vi "电子学自测试.vi"() -> ()   [LabVIEW 2017]
panel:
  in  "data  path":path=path "G:/rpc测试"
  out "appended path":path=path "D:/rpc测试/test_20260314_040925.txt"
  in  "filename":string="test"
  out "异常板卡":cluster{i32, i32}[](array[cluster])
  out "数字":i32=500
  out "当前累计":bool[][](array[boolean])
  out "当前Middle":bool[][](array[boolean])
  in  "停止":bool
  out "当前TDC":bool[](array[boolean])
  out "最终结果":bool[][][](array[boolean])
  out "trigger_rate":dbl[](array[numeric])=[-1.0, -1.0, -1.0, -1.0, -1.0, -1.0, -1.0, -1.0, -1.0, -1.0]
  out "error out":errorcluster
  out "TDC_ID":u64=2
  out "Middle ID":u64=1
  in  "TriggerRate":u8(ring)=2 items=["125Hz", "250Hz", "500Hz", "1000Hz", "2000Hz", "4000Hz", "5000Hz", "10000Hz", "20000Hz", "50000Hz"]
  in  "SoftTrigger":bool=TRUE
  in  "error in (no error)":errorcluster
  in  "address":string="10.3.173.20"
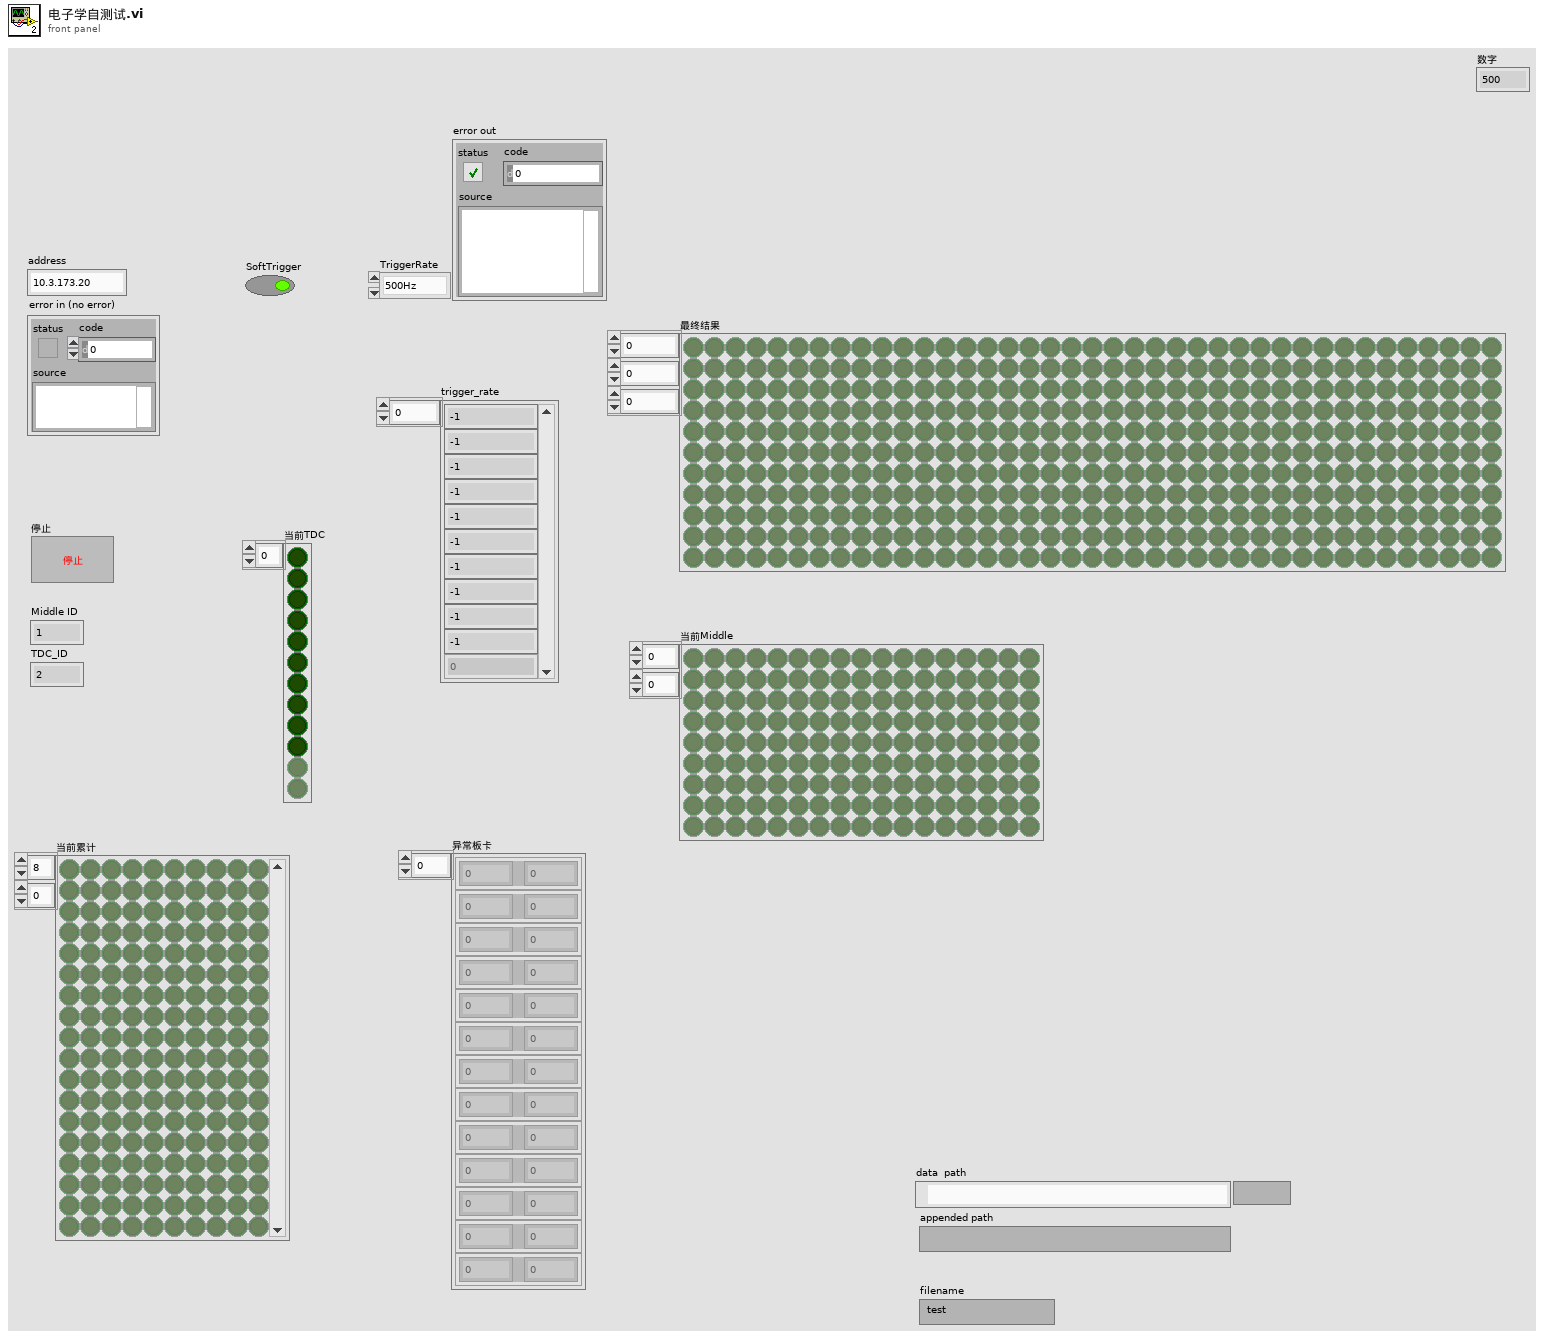
[diagram p1: front panel]
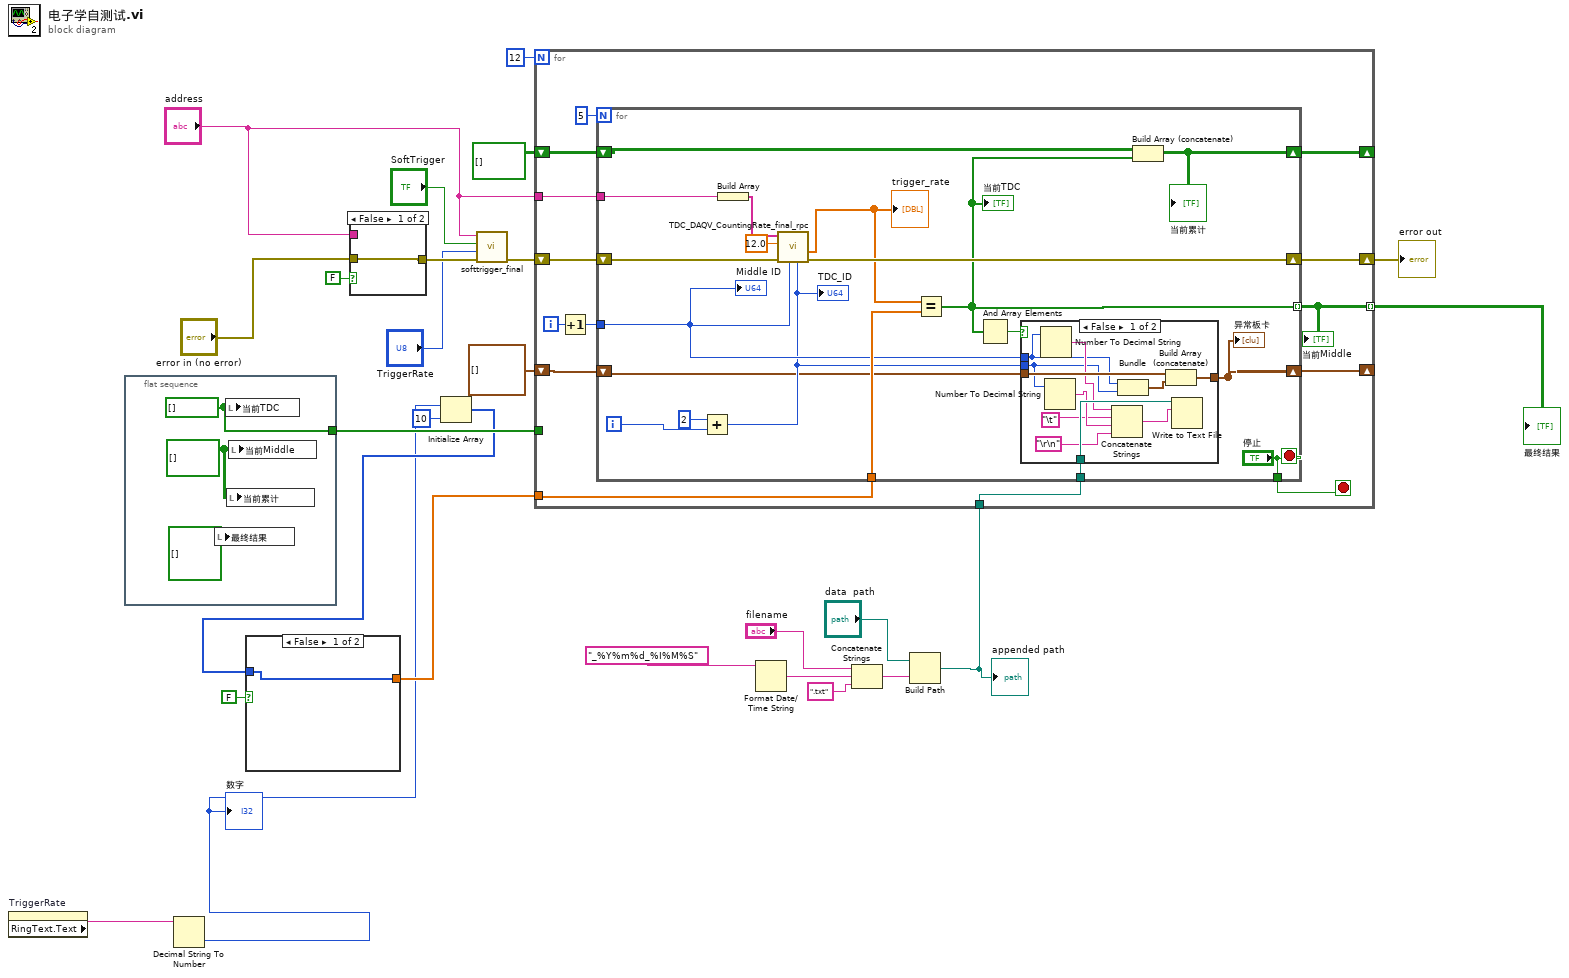
[diagram p0: block diagram]
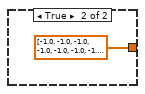
[diagram p2: hidden frame]
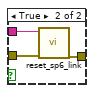
[diagram p4: hidden frame]
diagram:
  n1 = property on="TriggerRate" class="Ring (strict)"() -> ("RingText.Text"=w11:string)  [unwired: 2 in, 2 out]
  n2 = flat-sequence {
    tunnel: [w27] -> w14
    frame #0 {
      w29 = bool[][] [] ("当前Middle")
      w27 = bool[] [] ("当前TDC")
      n3 = local write "最终结果"(bool[][][] [] ("数组")) -> ()
      n4 = local write "当前TDC"(w27) -> ()
      n5 = local write "当前累计"(w29) -> ()
      n6 = local write "当前Middle"(w29) -> ()
    }
  }
  n7 = Decimal String To Number(string=w11) -> (number=w9:i32)  [unwired: 2 in, 1 out]
  "数字" <- w9
  n8 = case shown="False" FALSE {
    tunnel: "error in (no error)" -> [w30 w33]
    tunnel: [w30 w32] -> w25
    tunnel: "address" -> [_ w31]
    frame False {
    }
    frame True {
      n9 = call "reset_sp6_link.vi"("error in (no error)"=w33, "address"=w31) -> ("error out"=w32:errorcluster)  [unwired: 9 in]
    }
  }
  n10 = Initialize Array(w9, 10 ("维数大小")) -> (w12:i32[])
  n11 = case shown="False" FALSE {
    tunnel: [w34 dbl[] [-1.0, -1.0, -1.0, -1.0, -1.0, -1.0, -1.0, -1.0, -1.0, -1.0] ("rate_array")] -> w16
    tunnel: w12 -> [w34 _]
    frame False {
    }
    frame True {
    }
  }
  n12 = call "softtrigger_final.vi"("error in (no error)"=w25, "TriggerRate"="TriggerRate", "SoftTrigger"="SoftTrigger", "address"="address") -> ("error out"=w22:errorcluster)  [unwired: 7 in]
  n13 = Format Date/Time String(time format string (%c)="_%Y%m%d_%I%M%S") -> (date/time string=w6:string)  [unwired: 2 in]
  n14 = Concatenate Strings("filename", w6, ".txt") -> (w8:string)
  n15 = Build Path(base path="data  path", name or relative path=w8) -> (appended path=w3:path)
  "appended path" <- w3
  n16 = for {
    N: 12 -> [_]
    tunnel: "address" -> [w49]
    shift-right: [w47] -> w21
    shift-left: w22 -> [w48]
    tunnel: w16 -> [w45]
    tunnel: [w44] -> w18 mode=indexing
    shift-right: [w40] -> _
    shift-left: bool[][] [] -> [w39]
    tunnel: w14 -> [_]
    shift-right: [w38] -> _
    shift-left: cluster{i32, i32}[] [] -> [w37]
    tunnel: w3 -> [w36]
    i -> [w46]
    stop <- w41 stop-if-true
    n17 = Increment(x=w46) -> (x+1=w42:i32)
    n18 = for {
      N: 5 -> [_]
      tunnel: w49 -> [w68]
      shift-right: [w65] -> w47
      shift-left: w48 -> [w66]
      tunnel: w42 -> [w54]
      tunnel: w45 -> [w62]
      tunnel: [w56] -> w44 mode=indexing
      tunnel: ["停止"] -> w41
      shift-right: [w59] -> w40
      shift-left: w39 -> [w58]
      shift-right: [w50] -> w38
      shift-left: w37 -> [w52]
      tunnel: w36 -> [w51]
      i -> [w64]
      stop <- "停止" stop-if-true
      n19 = Add(x=2, y=w64) -> (x+y=w53:i32)
      "TDC_ID" <- w53
      n20 = Build Array(w68) -> (w67:string[])
      n21 = call "TDC_DAQV_CountingRate_final_rpc.vi"("TDC_ID"=w53, "Middle ID"=w54, "error in (no error)"=w66, "timeout"=12.0, "Array"=w67) -> ("error out"=w65:errorcluster, "trigger_rate"=w63:dbl[])  [unwired: 4 in, 1 out]
      "trigger_rate" <- w63
      n22 = Equal?(x=w63, y=w62) -> (x = y?=w56:bool[])
      "当前TDC" <- w56
      n23 = And Array Elements(Boolean array=w56) -> (logical AND=w55:bool)
      n24 = case shown="False" w55 {
        tunnel: w54 -> [w70 _]
        tunnel: w53 -> [w69 _]
        tunnel: w52 -> [w79 w80]
        tunnel: [w78 w80] -> w50
        tunnel: w51 -> [w76 _]
        frame False {
          n25 = Number To Decimal String(number=w70) -> (decimal integer string=w74:string)  [unwired: 1 in]
          n26 = Number To Decimal String(number=w69) -> (decimal integer string=w73:string)  [unwired: 1 in]
          n27 = Concatenate Strings(w74, "\t", w73, "\r\n") -> (w75:string)
          n28 = Bundle(w70, w69) -> (w77:cluster{i32, i32})  [unwired: 1 in]
          n29 = Build Array (concatenate)(w79, w77) -> (w78:cluster{i32, i32}[])
          n30 = Write to Text File(file (use dialog)=w76, text=w75) -> ()  [unwired: 2 in, 3 out]
        }
        frame True {
        }
      }
      "异常板卡" <- w50
      n31 = Build Array (concatenate)(w58, w56) -> (w59:bool[][])
      "当前累计" <- w59
      "Middle ID" <- w54
    }
    "当前Middle" <- w44
  }
  "error out" <- w21
  "最终结果" <- w18
